vi "FRCts20_WebMethods_Home_GET.vi"(10 "Debug":bool, 11 "httpRequestID":u32) -> (3 "error out":errorcluster)   [LabVIEW 2013, in "FRCts20_WebMethods.lvlib"]
uses:
  FRCts20_WebMethods.lvlib
  Backend/source/VI Source/FRCts20_Backend_API/FRCts20_Backend_API.lvlib
  Backend/source/VI Source/FRCts20_Backend_API/FRCts20_Backend_API_EventRoot.vi
  Backend/source/VI Source/FRCts20_Backend_API/FRCts20_Backend_API_Command_EventRoot.ctl
  ESP Engine/source/VI Source/FRCts20_EspEngine.lvlib
  Backend/source/VI Source/FRCts20_Backend_API/FRCts20_Backend_API_EventRoot.ctl
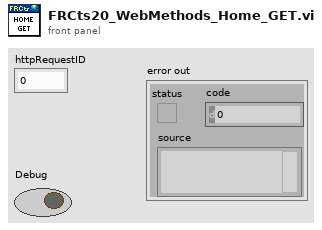
[diagram p1: front panel]
types:
  T1 = typedef "FRCts20_Backend_API.lvlib/FRCts20_Backend_API_EventRoot.ctl" = cluster{"Event":cluster{"Event Index":u32, "Event Name":string, "Start Time":timestamp, "End Time":timestamp, "OpenIssues":u8, "IsLive":bool}[], "APIReturn":string}
  T2 = typedef "FRCts20_Backend_API.lvlib/FRCts20_Backend_API_Command_EventRoot.ctl" = string
  T3 = typedef "FRCts20_EspEngine.lvlib/FRCts20_EspEngine_SearchBrowser.ctl" = cluster{"Event":cluster{"Event Index":u32, "Event Name":string, "Start Time":timestamp, "End Time":timestamp, "OpenIssues":u8, "IsLive":bool}[], "select-choice-software":string, "select-choice-location":string}
  T4 = cluster{"Event Index":u32, "Event Name":string, "Start Time":timestamp, "End Time":timestamp, "OpenIssues":u8, "IsLive":bool}[]
  T5 = typedef "FRCts20_EspEngine.lvlib/FRCts20_EspEngine_Universe.ctl" = cluster{"TeamsListLength":i16, "Teams":T6[], "LiveEventListLength":i16, "LiveEvents":T12[], "NonLiveEventListLength":i16, "NonLiveEvents":T12[], "OpenIssueCount":i16, "NotFoundStatus":bool}
  T6 = typedef "FRCts20_EspEngine.lvlib/FRCts20_EspEngine_Team.ctl" = cluster{"Team":T7, "RequestListLength":i16, "Requests":T10[]}
  T7 = typedef "FRCts20_WebMethods.lvlib/FRCts20_WebMethods_ctl_singleTeam.ctl" = cluster{"Events":string[], "Robot Name":string, "Kinect":bool, "Vision":bool, "Can":bool, "Tags":string, "Avatar URL":string, "Team":T8, "SWType":T9}
  T8 = typedef "FRCts20_WebMethods.lvlib/FRCts20_WebMethods_ctl_teamIdentifier.ctl" = cluster{"Team Nickname":string, "Team Number ":u32, "UniqueId":u32}
  T9 = typedef "FRCts20_Backend_API.lvlib/FRCts20_Backend_API_SW.ctl" = string
  T10 = typedef "FRCts20_WebMethods.lvlib/FRCts20_WebMethods_ctl_request.ctl" = cluster{"Event":string, "Description":string, "Status":T11, "Open Date":string, "Last Update":string, "Close Date":string, "UniqueId":i32, "Team":cluster{"Team Nickname":string, "Team Number ":i32, "UniqueId":i32}, "Comments":cluster{"Request Number":dbl, "Text":string, "Author":string, "IsSolution":bool, "Team":cluster{"Team Nickname":string, "Team Identifier ":dbl}, "UniqueId":i32}[]}
  T11 = typedef "FRCts20_Backend_API.lvlib/FRCts20_Backend_API_Status.ctl" = enum16{"Open", "In Work", "Closed"}
  T12 = typedef "FRCts20_EspEngine.lvlib/FRCts20_EspEngine_Event.ctl" = cluster{"Single Event":T13, "EventOpenIssueCount":i16, "Requests":cluster{"RequestId":i32, "Request Description":string, "Team Number":i32}[], "ClosedRequests":cluster{"RequestId":i32, "Request Description":string, "Team Number":i32}[], "NotFoundStatus":bool}
  T13 = typedef "FRCts20_WebMethods.lvlib/FRCts20_WebMethods_ctl_singleEvent.ctl" = cluster{"Team":T8[], "Issue Count":i32, "Location":string, "Start Date ":timestamp}
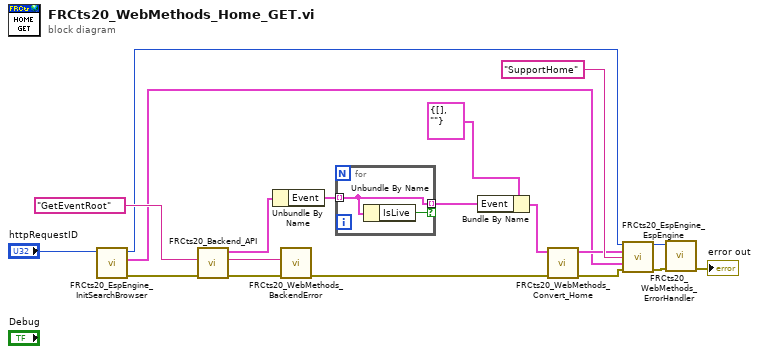
[diagram p0: block diagram]
diagram:
  n1 = call "FRCts20_EspEngine_InitSearchBrowser.vi"("httpRequestID"="httpRequestID") -> ("error out"=w4:errorcluster, "SearchBrowser"=w1:T3, "httpRequestID out"=w2:u32)  [unwired: 8 in]
  n2 = call-poly "FRCts20_Backend_API.vi"("error in (no error)"=w4, "Message"=T2 "GetEventRoot") -> ("error out"=w14:errorcluster, "Status"=w17:string, "EventRoot Out"=w12:T1)  [unwired: 7 in]
  n3 = Unbundle By Name(w12) -> ("Event"=w15:T4)
  n4 = call "FRCts20_WebMethods_BackendError.vi"("error in (no error)"=w14, "Status"=w17) -> ("error out"=w5:errorcluster)  [unwired: 8 in, 1 out]
  n5 = for {
    tunnel: w15 -> [w21] mode=indexing
    tunnel: [w21] -> w10 mode=indexing if=w20
    n6 = Unbundle By Name(w21) -> ("IsLive"=w20:bool)
  }
  n7 = Bundle By Name(cluster=T1 {"Event"=[], "APIReturn"=""} ("EventRoot Out"), "Event"=w10) -> (w9:T1)
  n8 = call "FRCts20_WebMethods_Convert_Home.vi"("error in (no error)"=w5, "EventRoot Out"=w9) -> ("error out"=w7:errorcluster, "Universe"=w6:T5)  [unwired: 8 in]
  n9 = call "FRCts20_EspEngine_EspEngine.vi"("httpRequestID"=w2, "Cluster"=w6, "Page"="SupportHome", "SearchBrowser"=w1, "error in (no error)"=w7) -> ("httpRequestID out"=w18:u32, "error out"=w19:errorcluster)  [unwired: 9 in]
  n10 = call "FRCts20_WebMethods_ErrorHandler.vi"("error in"=w19, "httpRequestID"=w18) -> ("error out"=→"error out":errorcluster)  [unwired: 9 in]
